vi "Check start of line for constant.vi"(10 "Constant to check start of line":string, 11 "Line":string) -> (3 "Does it start with constant?":bool)   [LabVIEW 2013]
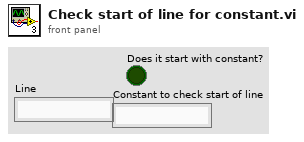
[diagram p1: front panel]
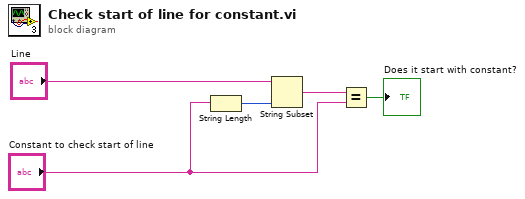
[diagram p0: block diagram]
diagram:
  n1 = String Length(string="Constant to check start of line") -> (length=w2:i32)
  n2 = String Subset(string="Line", length (rest)=w2) -> (substring=w5:string)  [unwired: 1 in]
  n3 = Equal?(x=w5, y="Constant to check start of line") -> (x = y?=→"Does it start with constant?":bool)
